vi "GetDevInfo.vi"(8 "错误输入（无错误）":errorcluster, 10 "Model":string, 11 "ConfigFile":path) -> (0 "error out":errorcluster caption="错误输出", 1 "需要掃描的":T2(array[cluster]), 2 "所有的":cluster{i32, bool}[](array[cluster]))   [LabVIEW 2012]
uses:
  Fun/Dev/SupportVi/DevState.ctl
  <vilib>/Utility/config.llb/Read Key (U32).vi
  <vilib>/Utility/config.llb/Read Key (String).vi
  <vilib>/Utility/config.llb/NI_LVConfig.lvlib
  Fun/Dev/DevControl.lvclass
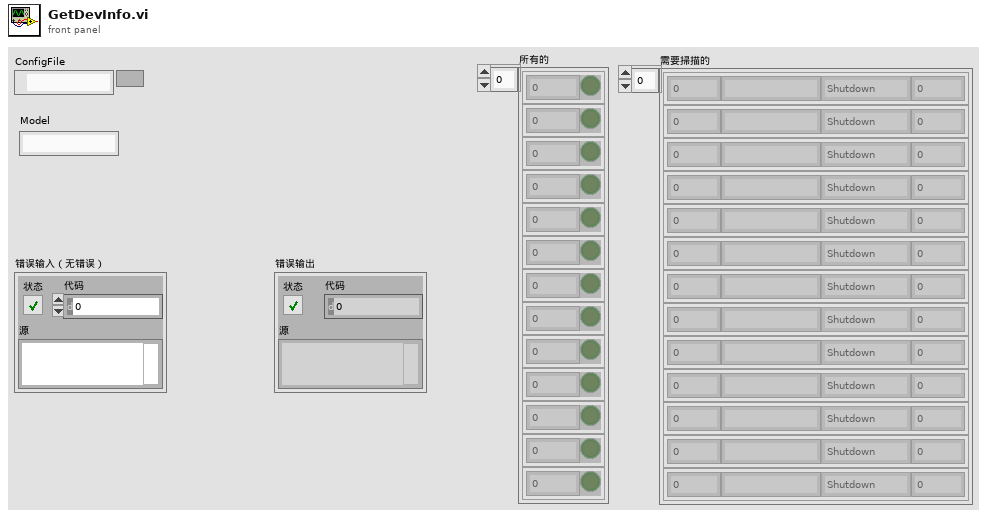
[diagram p1: front panel]
types:
  T1 = typedef "DevControl.lvclass/DevState.ctl" = enum16{"Shutdown", "PASS", "FAIL", "Idle", "Noresponse"}
  T2 = cluster{"Addr":i32, "name":string, "State":T1, "Retry":i32}[]
  T3 = typedef "NI_LVConfig.lvlib/Config Data RefNum.ctl" = refnum<k1>
  T4 = cluster{i32, "trimmed string":string, "ÑbÖÃ î‘B":T1, i32}
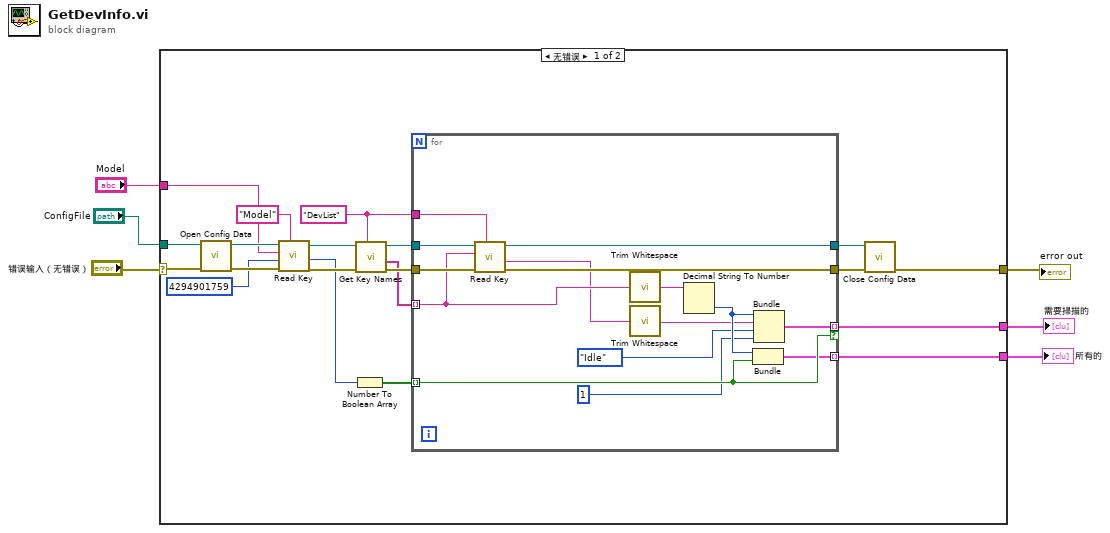
[diagram p0: block diagram]
diagram:
  n1 = case shown="无错误" "错误输入（无错误）" {
    selector: "错误输入（无错误）" -> [w25 w42]
    tunnel: "ConfigFile" -> [w26 _]
    tunnel: "Model" -> [w22 _]
    tunnel: [w11 _] -> w1
    tunnel: [w10 _] -> w3
    tunnel: [w7 w42] -> w2
    frame No Error {
      w12 = "DevList" ("section")
      n2 = call <vilib>:"Open Config Data.vi"("error in (no error)"=w25, "configuration file path"=w26) -> ("error out"=w23:errorcluster, "refnum"=w24:T3)  [unwired: 7 in, 1 out]
      n3 = call-poly <vilib>:"Read Key.vi"("section"="Model", "error in (no error)"=w23, "default value"=u32 4294901759, "key"=w22, "refnum"=w24) -> ("error out"=w19:errorcluster, "value"=w15:u32, "refnum out"=w20:T3)  [unwired: 3 in, 1 out]
      n4 = Number To Boolean Array(number=w15) -> (Boolean array=w13:bool[])
      n5 = call <vilib>:"Get Key Names.vi"("section"=w12, "error in (no error)"=w19, "refnum"=w20) -> ("error out"=w18:errorcluster, "key names"=w16:string[], "refnum out"=w17:T3)  [unwired: 5 in, 1 out]
      n6 = for {
        tunnel: w18 -> [w40]
        tunnel: w17 -> [w41]
        tunnel: w16 -> [w29] mode=indexing
        tunnel: w13 -> [w36] mode=indexing
        tunnel: w12 -> [w39]
        tunnel: [w38] -> w11 mode=indexing if=w36
        tunnel: [w35] -> w10 mode=indexing
        tunnel: [w34] -> w9
        tunnel: [w31] -> w8
        n7 = call-poly <vilib>:"Read Key.vi"("section"=w39, "error in (no error)"=w40, "key"=w29, "refnum"=w41) -> ("error out"=w34:errorcluster, "value"=w27:string, "refnum out"=w31:T3)  [unwired: 4 in, 1 out]
        n8 = call <vilib>:"Trim Whitespace.vi"("string"=w29) -> ("trimmed string"=w30:string)  [unwired: 1 in]
        n9 = call <vilib>:"Trim Whitespace.vi"("string"=w27) -> ("trimmed string"=w28:string)  [unwired: 1 in]
        n10 = Decimal String To Number(string=w30) -> (number=w37:i32)  [unwired: 2 in, 1 out]
        n11 = Bundle(w37, w36) -> (w35:cluster{i32, bool})  [unwired: 1 in]
        n12 = Bundle(w37, "trimmed string"=w28, "ÑbÖÃ î‘B"=DevState."Idle", 1) -> (w38:T4)  [unwired: 1 in]
      }
      n13 = call <vilib>:"Close Config Data.vi"("error in (no error)"=w9, "refnum"=w8) -> ("error out"=w7:errorcluster)  [unwired: 8 in, 1 out]
    }
    frame Error {
    }
  }
  "error out" <- w2
  "所有的" <- w3
  "需要掃描的" <- w1
